vi "Add View.vi"(0 "Controller Actor in":refnum<class "Controller Actor.lvclass">, 1 "View Actor":refnum<class "View Actor.lvclass">, 2 "Exclude From Broadcast (F)":bool, 3 "Paused (F)":bool, 4 "Receive Only (F)":bool, 5 "error in (no error)":errorcluster) -> (14 "Controller Actor out":refnum<class "Controller Actor.lvclass">, 16 "View Enqueuer":refnum<class "Message Enqueuer.lvclass">, 19 "error out":errorcluster)   [LabVIEW 2023, in "Event Actors.lvlib" / "Controller Actor.lvclass"]
doc: "Starts a View Actor with following settings:\n\n<b>Exclude From Broadcast</b>: message originating form another view will not be broadcasted to the view being cosidered\n<b>Paused</b>: the view will not send events and will not receive them anymore\n<b>Receive only</b>: The view will receive events but not send any"
uses:
  Controller Actor.lvclass
  C:/Program Files/National Instruments/LabVIEW 2023/vi.lib/ActorFramework/Actor/Actor.lvclass
  View Actor/View Actor.lvclass
  <vilib>/ActorFramework/Message Enqueuer/Message Enqueuer.lvclass
  View Details.ctl
  View Actor/View Actor.lvclass/View Actor.ctl
  Controller Actor.lvclass/Controller Actor.ctl
  <vilib>/ActorFramework/Actor/Actor.lvclass/Actor.ctl
  <vilib>/ActorFramework/Message Enqueuer/Message Enqueuer.lvclass/Message Enqueuer.ctl
  View Actor Messages/Write Controller Actor Enqueuer Msg/Write Controller Actor Enqueuer Msg.lvclass/Write Controller Actor Enqueuer Msg.ctl
  View Actor/properties/Read Name.vi
  View Actor/properties/Write Paused.vi
  View Actor/properties/Write Receive Only.vi
  <vilib>/ActorFramework/Message Enqueuer/Init from Existing Queue.vi
  <vilib>/ActorFramework/Message Enqueuer/Enqueue.vi
  View Actor Messages/Write Controller Actor Enqueuer Msg/Write Controller Actor Enqueuer Msg.lvclass
  C:/Program Files/National Instruments/LabVIEW 2023/vi.lib/ActorFramework/Message/Message.lvclass
  <vilib>/Utility/LVClass/Get LV Class Name.vi
  <resource>/AFDebug/Generate Trace for Message.vi
  <vilib>/ActorFramework/Message Priority Queue/Priority Enqueue.vi
  <vilib>/ActorFramework/Actor/Actor.lvclass
  C:/Projects/Shared Libraries/Event Actors/Controller Actor/Controller Actor.lvclass
  C:/Projects/Hardware Controller/Source/LSI Hardware Controller/View Interface/IView.lvclass
  C:/Projects/Shared Libraries/Event Actors/View Actor/View Actor.lvclass
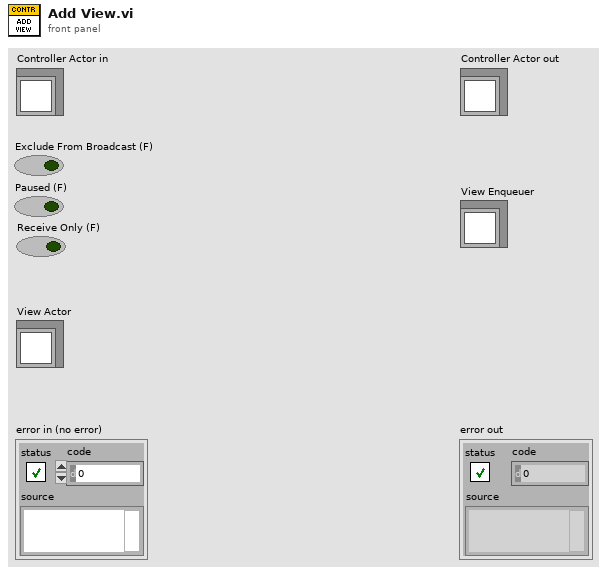
[diagram p1: front panel]
types:
  T1 = typedef "Event Actors.lvlib/Controller Actor.lvclass/View Details.ctl" = cluster{"Exclude From Broadcast":bool, "Receive Only":bool, "Paused":bool, "View Enqueuer":refnum<class "Message Enqueuer.lvclass">}
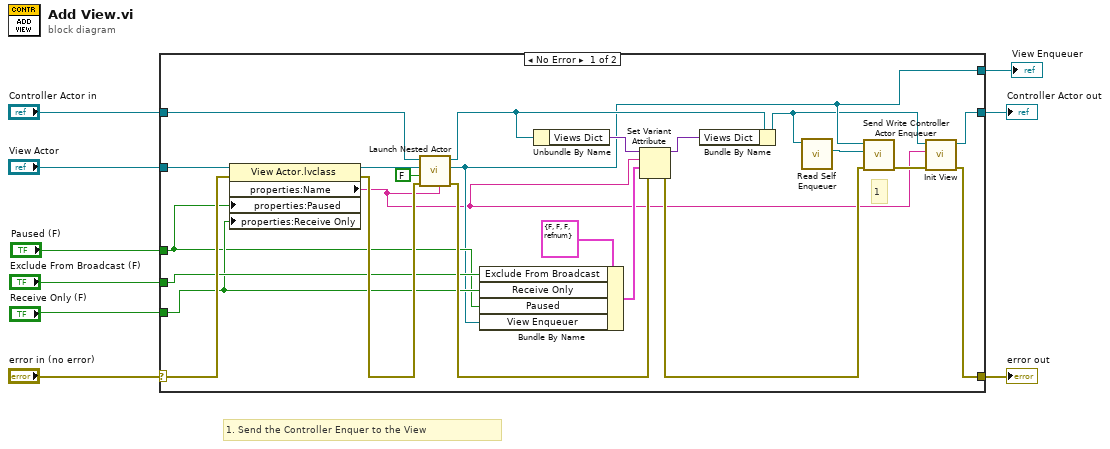
[diagram p0: block diagram]
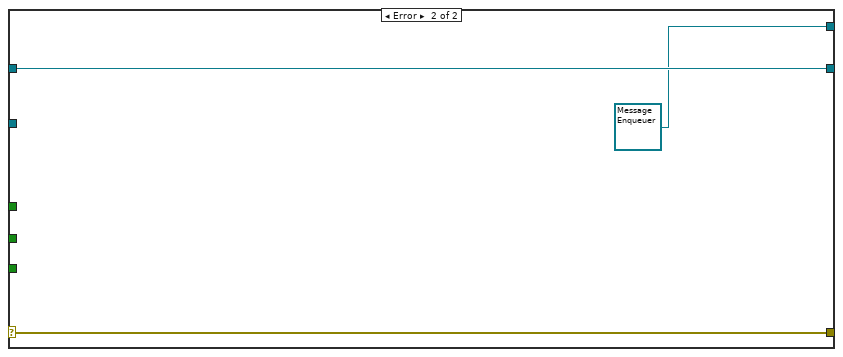
[diagram p2: hidden frame]
diagram:
  # "1. Send the Controller Enquer to the View"
  n1 = case shown="No Error" "error in (no error)" {
    selector: "error in (no error)" -> [w24 w35]
    tunnel: [w11 w35] -> w8
    tunnel: [w13 w34] -> w6
    tunnel: "Controller Actor in" -> [w28 w34]
    tunnel: "View Actor" -> [w29 _]
    tunnel: "Paused (F)" -> [w16 _]
    tunnel: "Exclude From Broadcast (F)" -> [w18 _]
    tunnel: "Receive Only (F)" -> [w17 _]
    tunnel: [w15 refnum<class "Message Enqueuer.lvclass"> refnum ("Nested Actor's Enqueuer")] -> w1
    frame No Error {
      # "1"
      n2 = property class="View Actor.lvclass"(reference=w29, error in=w24, "properties:Paused"=w16, "properties:Receive Only"=w17) -> (reference out=w25:refnum<class "View Actor.lvclass">, error out=w23:errorcluster, "properties:Name"=w10:string)
      n3 = call <vilib>:"Launch Nested Actor.vi"("Debug Alias"=w10, "error in (no error)"=w23, "Auto-stop? (T)"=FALSE, "Nested Actor"=w25, "Caller Actor in"=w28) -> ("error out"=w30:errorcluster, "Nested Actor's Enqueuer"=w15:refnum<class "Message Enqueuer.lvclass">, "Caller Actor out"=w27:refnum<class "Controller Actor.lvclass">)  [unwired: 4 in]
      n4 = Bundle By Name(cluster=T1 {"Exclude From Broadcast"=FALSE, "Receive Only"=FALSE, "Paused"=FALSE, "View Enqueuer"=refnum} ("Sink Settings"), "Exclude From Broadcast"=w18, "Receive Only"=w17, "Paused"=w16, "View Enqueuer"=w15) -> (w19:T1)
      n5 = Unbundle By Name(w27) -> ("Views Dict"=w32:variant)
      n6 = Set Variant Attribute(Variant=w32, name=w10, value=w19, error in=w30) -> (Variant out=w31:variant, error out=w21:errorcluster)  [unwired: 1 out]
      n7 = Bundle By Name(cluster=w27, "Views Dict"=w31) -> (w14:refnum<class "Controller Actor.lvclass">)
      n8 = call <vilib>:"Read Self Enqueuer.vi"("Actor"=w14) -> ("Self Enqueuer"=w22:refnum<class "Message Enqueuer.lvclass">)  [unwired: 10 in]
      n9 = call "Send Write Controller Actor Enqueuer.vi"("error in (no error)"=w21, "Controller Actor Enqueuer"=w22, "Message Enqueuer in"=w15) -> ("error out"=w12:errorcluster)  [unwired: 7 in, 1 out]
      n10 = call-dynamic "Init View.vi"("error in (no error)"=w12, "View Name"=w10, "Controller Actor in"=w14) -> ("error out"=w11:errorcluster, "Controller Actor out"=w13:refnum<class "Controller Actor.lvclass">)  [unwired: 7 in]
    }
    frame Error {
    }
  }
  "error out" <- w8
  "Controller Actor out" <- w6
  "View Enqueuer" <- w1
